vi "ControlMotorParam.vi"(3 "电机":enum16{"Z", "Y", "X", "发散角", "俯仰", "旋转"}(ring)) -> (1 "轴电机参数输出":T1)   [LabVIEW 2018]
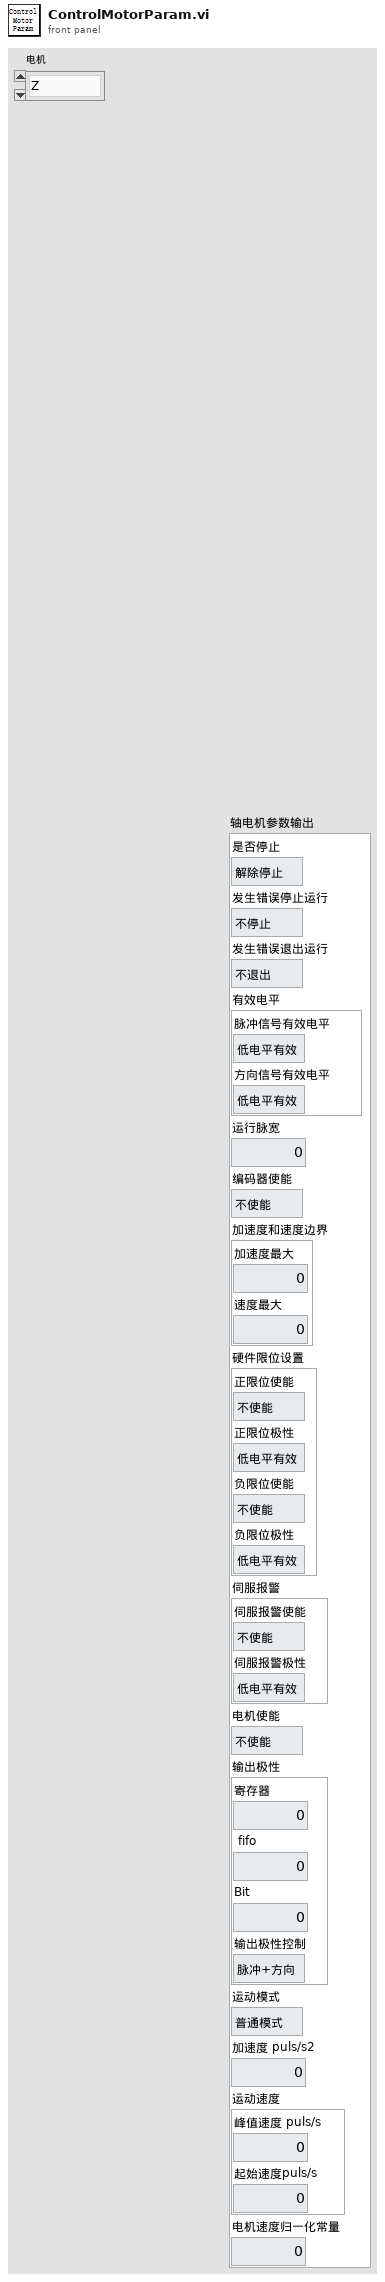
[diagram p1: front panel]
types:
  T1 = cluster{"是否停止":enum16{"解除停止", "停止"}, "发生错误停止运行":enum16{"不停止", "停止"}, "发生错误退出运行":enum16{"不退出", "退出"}, "有效电平":cluster{"脉冲信号有效电平":enum16{"低电平有效", "高电平有效"}, "方向信号有效电平 ":enum16{"低电平有效", "高电平有效"}}, "运行脉宽":i32, "编码器使能":enum16{"不使能", "使能"}, "加速度和速度边界":cluster{"加速度最大":i32, "速度最大":i32}, "硬件限位设置":cluster{"正限位使能":enum16{"不使能", "使能"}, "正限位极性":enum16{"低电平有效", "高电平有效"}, "负限位使能 ":enum16{"不使能", "使能"}, "负限位极性 ":enum16{"低电平有效", "高电平有效"}}, "伺服报警":cluster{"伺服报警使能":enum16{"不使能", "使能"}, "伺服报警极性":enum16{"低电平有效", "高电平有效"}}, "电机使能":enum16{"不使能", "使能"}, "输出极性":cluster{"寄存器":u32, " fifo":u32, "Bit":u32, "输出极性控制":enum16{"脉冲+方向", "正负脉冲"}}, "运动模式":enum16{"普通模式", "跟踪模式"}, "加速度 puls/s2":i32, "运动速度":cluster{"峰值速度 puls/s":i32, "起始速度puls/s":i32}, "电机速度归一化常量":dbl}
  T2 = cluster{"是否停止":enum16{"解除停止", "停止"}, "发生错误停止运行":enum16{"不停止", "停止"}, "发生错误退出运行":enum16{"不退出", "退出"}, "有效电平":cluster{"脉冲信号有效电平":enum16{"低电平有效", "高电平有效"}, "方向信号有效电平 ":enum16{"低电平有效", "高电平有效"}}, "运行脉宽":i32, "编码器使能":enum16{"不使能", "使能"}, "加速度和速度边界":cluster{"加速度最大":i32, "速度最大":i32}, "硬件限位设置":cluster{"正限位使能":enum16{"不使能", "使能"}, "正限位极性":enum16{"低电平有效", "高电平有效"}, "负限位使能 ":enum16{"不使能", "使能"}, "负限位极性 ":enum16{"低电平有效", "高电平有效"}}, "伺服报警":cluster{"伺服报警使能":enum16{"不使能", "使能"}, "伺服报警极性":enum16{"低电平有效", "高电平有效"}}, "电机使能":enum16{"不使能", "使能"}, "输出极性":cluster{"寄存器":u32, " fifo":u32, "Bit":u32, "输出极性控制":enum16{"脉冲+方向", "正负脉冲"}}, "运动模式":enum16{"普通模式", "跟踪模式"}, "加速度 puls/s2":i32, "运动速度":cluster{"峰值速度 puls/s":i32, "起始速度puls/s":i32}, "电机速度归一化常量":dbl}[]
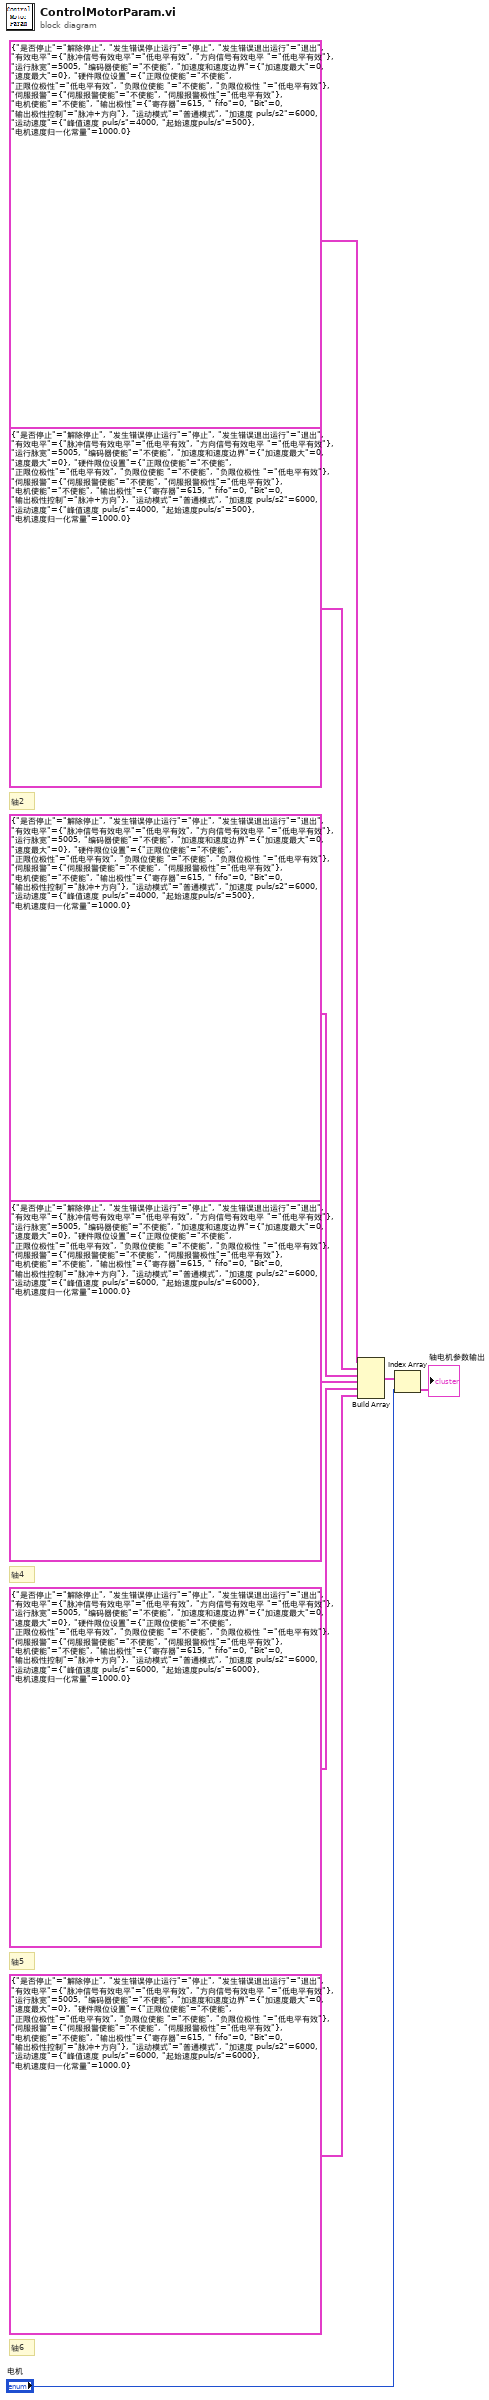
[diagram p0: block diagram]
diagram:
  # "轴6"
  # "轴5"
  # "轴4"
  # "轴3"
  # "轴2"
  # "轴1"
  n1 = Build Array(T1 {"是否停止"=enum."解除停止", "发生错误停止运行"=enum."停止", "发生错误退出运行"=enum."退出", "有效电平"={"脉冲信号有效电平"=enum."低电平有效", "方向信号有效电平 "=enum."低电平有效"}, "运行脉宽"=5005, "编码器使能"=enum."不使能", "加速度和速度边界"={"加速度最大"=0, "速度最大"=0}, "硬件限位设置"={"正限位使能"=enum."不使能", "正限位极性"=enum."低电平有效", "负限位使能 "=enum."不使能", "负限位极性 "=enum."低电平有效"}, "伺服报警"={"伺服报警使能"=enum."不使能", "伺服报警极性"=enum."低电平有效"}, "电机使能"=enum."不使能", "输出极性"={"寄存器"=615, " fifo"=0, "Bit"=0, "输出极性控制"=enum."脉冲+方向"}, "运动模式"=enum."普通模式", "加速度 puls/s2"=6000, "运动速度"={"峰值速度 puls/s"=4000, "起始速度puls/s"=500}, "电机速度归一化常量"=1000.0} ("轴参数"), T1 {"是否停止"=enum."解除停止", "发生错误停止运行"=enum."停止", "发生错误退出运行"=enum."退出", "有效电平"={"脉冲信号有效电平"=enum."低电平有效", "方向信号有效电平 "=enum."低电平有效"}, "运行脉宽"=5005, "编码器使能"=enum."不使能", "加速度和速度边界"={"加速度最大"=0, "速度最大"=0}, "硬件限位设置"={"正限位使能"=enum."不使能", "正限位极性"=enum."低电平有效", "负限位使能 "=enum."不使能", "负限位极性 "=enum."低电平有效"}, "伺服报警"={"伺服报警使能"=enum."不使能", "伺服报警极性"=enum."低电平有效"}, "电机使能"=enum."不使能", "输出极性"={"寄存器"=615, " fifo"=0, "Bit"=0, "输出极性控制"=enum."脉冲+方向"}, "运动模式"=enum."普通模式", "加速度 puls/s2"=6000, "运动速度"={"峰值速度 puls/s"=4000, "起始速度puls/s"=500}, "电机速度归一化常量"=1000.0} ("轴参数"), T1 {"是否停止"=enum."解除停止", "发生错误停止运行"=enum."停止", "发生错误退出运行"=enum."退出", "有效电平"={"脉冲信号有效电平"=enum."低电平有效", "方向信号有效电平 "=enum."低电平有效"}, "运行脉宽"=5005, "编码器使能"=enum."不使能", "加速度和速度边界"={"加速度最大"=0, "速度最大"=0}, "硬件限位设置"={"正限位使能"=enum."不使能", "正限位极性"=enum."低电平有效", "负限位使能 "=enum."不使能", "负限位极性 "=enum."低电平有效"}, "伺服报警"={"伺服报警使能"=enum."不使能", "伺服报警极性"=enum."低电平有效"}, "电机使能"=enum."不使能", "输出极性"={"寄存器"=615, " fifo"=0, "Bit"=0, "输出极性控制"=enum."脉冲+方向"}, "运动模式"=enum."普通模式", "加速度 puls/s2"=6000, "运动速度"={"峰值速度 puls/s"=4000, "起始速度puls/s"=500}, "电机速度归一化常量"=1000.0} ("轴参数"), T1 {"是否停止"=enum."解除停止", "发生错误停止运行"=enum."停止", "发生错误退出运行"=enum."退出", "有效电平"={"脉冲信号有效电平"=enum."低电平有效", "方向信号有效电平 "=enum."低电平有效"}, "运行脉宽"=5005, "编码器使能"=enum."不使能", "加速度和速度边界"={"加速度最大"=0, "速度最大"=0}, "硬件限位设置"={"正限位使能"=enum."不使能", "正限位极性"=enum."低电平有效", "负限位使能 "=enum."不使能", "负限位极性 "=enum."低电平有效"}, "伺服报警"={"伺服报警使能"=enum."不使能", "伺服报警极性"=enum."低电平有效"}, "电机使能"=enum."不使能", "输出极性"={"寄存器"=615, " fifo"=0, "Bit"=0, "输出极性控制"=enum."脉冲+方向"}, "运动模式"=enum."普通模式", "加速度 puls/s2"=6000, "运动速度"={"峰值速度 puls/s"=6000, "起始速度puls/s"=6000}, "电机速度归一化常量"=1000.0} ("轴参数"), T1 {"是否停止"=enum."解除停止", "发生错误停止运行"=enum."停止", "发生错误退出运行"=enum."退出", "有效电平"={"脉冲信号有效电平"=enum."低电平有效", "方向信号有效电平 "=enum."低电平有效"}, "运行脉宽"=5005, "编码器使能"=enum."不使能", "加速度和速度边界"={"加速度最大"=0, "速度最大"=0}, "硬件限位设置"={"正限位使能"=enum."不使能", "正限位极性"=enum."低电平有效", "负限位使能 "=enum."不使能", "负限位极性 "=enum."低电平有效"}, "伺服报警"={"伺服报警使能"=enum."不使能", "伺服报警极性"=enum."低电平有效"}, "电机使能"=enum."不使能", "输出极性"={"寄存器"=615, " fifo"=0, "Bit"=0, "输出极性控制"=enum."脉冲+方向"}, "运动模式"=enum."普通模式", "加速度 puls/s2"=6000, "运动速度"={"峰值速度 puls/s"=6000, "起始速度puls/s"=6000}, "电机速度归一化常量"=1000.0} ("轴参数"), T1 {"是否停止"=enum."解除停止", "发生错误停止运行"=enum."停止", "发生错误退出运行"=enum."退出", "有效电平"={"脉冲信号有效电平"=enum."低电平有效", "方向信号有效电平 "=enum."低电平有效"}, "运行脉宽"=5005, "编码器使能"=enum."不使能", "加速度和速度边界"={"加速度最大"=0, "速度最大"=0}, "硬件限位设置"={"正限位使能"=enum."不使能", "正限位极性"=enum."低电平有效", "负限位使能 "=enum."不使能", "负限位极性 "=enum."低电平有效"}, "伺服报警"={"伺服报警使能"=enum."不使能", "伺服报警极性"=enum."低电平有效"}, "电机使能"=enum."不使能", "输出极性"={"寄存器"=615, " fifo"=0, "Bit"=0, "输出极性控制"=enum."脉冲+方向"}, "运动模式"=enum."普通模式", "加速度 puls/s2"=6000, "运动速度"={"峰值速度 puls/s"=6000, "起始速度puls/s"=6000}, "电机速度归一化常量"=1000.0} ("轴参数")) -> (w3:T2)
  n2 = Index Array(array=w3, index="电机") -> (element=→"轴电机参数输出":T1)
